vi "AlliGator Enforce Lifetime Positivity.vi"(11 "Constraints in":T1[](array[typedef]) {"Max Value" format="%#.3g"; "Min Value" format="%#.3g"}) -> (3 "Constraints out":T1[](array[typedef]) {"Max Value" format="%#.3g"; "Min Value" format="%#.3g"})   [LabVIEW 2021, in "AlliGator Decay Analysis.lvlib" / "AlliGator Decay Fit.lvlib"]
doc: "Constrains lifetime parameters to be positive (replacing them by zero otherwise)."
uses:
  AlliGator Decay Fit.lvlib
  AlliGator Decay Fit Parameter Constraints 2.ctl
  Fits/IRF(X)PSED/Decay Fit Parameters In List.ctl
  Fits/Fits.lvlib
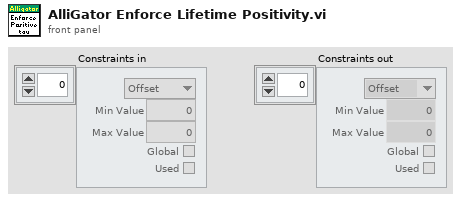
[diagram p1: front panel]
types:
  T1 = typedef "AlliGator Decay Analysis.lvlib/AlliGator Decay Fit.lvlib/AlliGator Decay Fit Parameter Constraints 2.ctl" = cluster{"Fit Parameter":T2, "Min Value":dbl, "Max Value":dbl, "Global":bool, "Used":bool}
  T2 = typedef "Fits.lvlib/Decay Fit Parameters In List.ctl" = enum16{"Offset", "Baseline", "A_1", "tau_1", "A_2", "tau_2"}
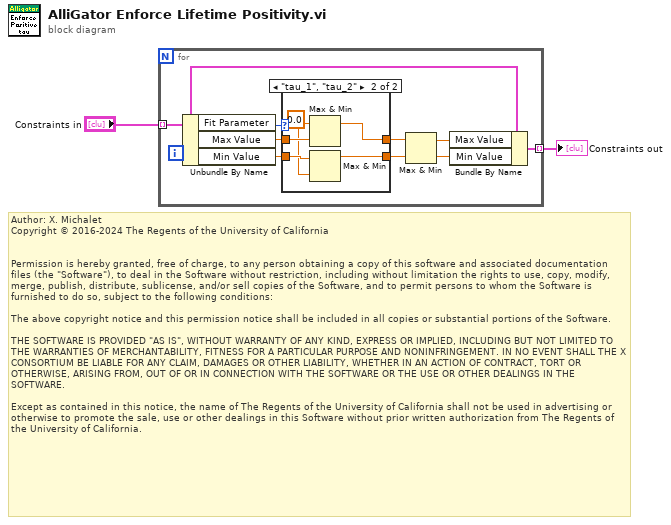
[diagram p0: block diagram]
diagram:
  # "Author: X. Michalet\nCopyright © 2016-2024 The Regents of the University of California\n \n\nPermission is hereby granted, free of charge, to any person obtaining a copy of this software and associated documentation files (the \"Software\"), to deal in the Software without restriction, including without limitation the rights to use, copy, modify, merge, publish, distribute, sublicense, and/or sell copies of the Software, and to permit persons to whom the Software is furnished to do so, subject to the following conditions:\n\nThe above copyright notice and this permission notice shall be included in all copies or substantial portions of the Software.\n\nTHE SOFTWARE IS PROVIDED \"AS IS\", WITHOUT WARRANTY OF ANY KIND, EXPRESS OR IMPLIED, INCLUDING BUT NOT LIMITED TO THE WARRANTIES OF MERCHANTABILITY, FITNESS FOR A PARTICULAR PURPOSE AND NONINFRINGEMENT. IN NO EVENT SHALL THE X CONSORTIUM BE LIABLE FOR ANY CLAIM, DAMAGES OR OTHER LIABILITY, WHETHER IN AN ACTION OF CONTRACT, TORT OR OTHERWISE, ARISING FROM, OUT OF OR IN CONNECTION WITH THE SOFTWARE OR THE USE OR OTHER DEALINGS IN THE SOFTWARE.\n\nExcept as contained in this notice, the name of The Regents of the University of California shall not be used in advertising or otherwise to promote the sale, use or other dealings in this Software without prior written authorization from The Regents of the University of California."
  n1 = for {
    tunnel: "Constraints in" -> [w9] mode=indexing
    tunnel: [w3] -> w1 mode=indexing
    n2 = Unbundle By Name(w9) -> ("Fit Parameter"=w11:T2, "Max Value"=w10:dbl, "Min Value"=w8:dbl)
    n3 = case shown="\"tau_1\", \"tau_2\"" w11 {
      tunnel: w10 -> [w13 w18]
      tunnel: w8 -> [w12 w17]
      tunnel: [w13 w15] -> w7
      tunnel: [w12 w14] -> w6
      frame "Offset", Default {
      }
      frame "tau_1", "tau_2" {
        w16 = 0.0 ("y")
        n4 = Max & Min(x=w16, y=w18) -> (max(x,y)=w15:dbl)  [unwired: 1 out]
        n5 = Max & Min(x=w17, y=w16) -> (max(x,y)=w14:dbl)  [unwired: 1 out]
      }
    }
    n6 = Max & Min(x=w7, y=w6) -> (max(x,y)=w5:dbl, min(x,y)=w4:dbl)
    n7 = Bundle By Name(cluster=w9, "Max Value"=w5, "Min Value"=w4) -> (w3:T1)
  }
  "Constraints out" <- w1
